vi "Find Path with Astar.vi"(8 "error in (no error)":errorcluster, 9 "goal node":cluster{"X":i32, "Y":i32}={"X"=32, "Y"=32}, 10 "start node":cluster{"X":i32, "Y":i32}={"X"=3, "Y"=3}, 11 "map reference in":refnum<data-value>) -> (1 "error out":errorcluster, 2 "intensity values":dbl[][](array[numeric]), 3 "map reference out":refnum<data-value>, 4 "y coordinates":i32[](array[numeric]), 6 "x coordinates":i32[](array[numeric]))   [LabVIEW 2017]
uses:
  <vilib>/robotics/Navigation/shared/WorldMap/OccupancyGridWorldMap/NI_Robotics_OccupancyGridWorldMap.lvclass
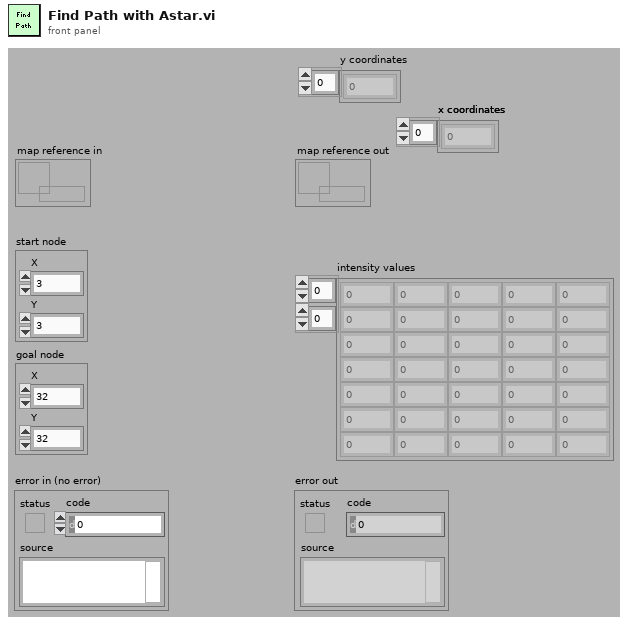
[diagram p1: front panel]
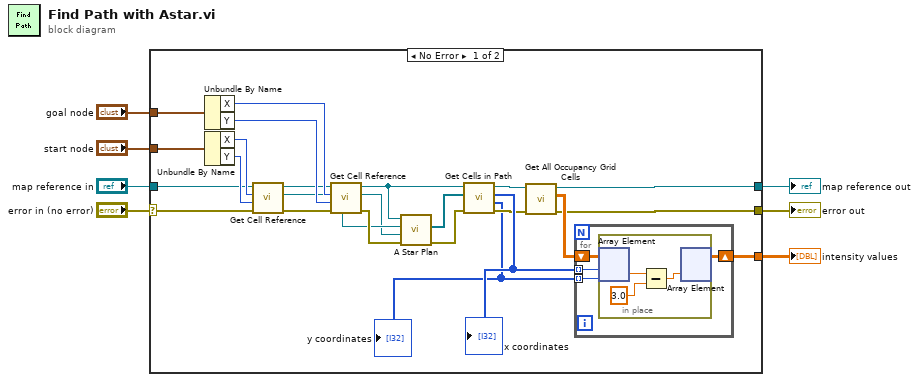
[diagram p0: block diagram]
diagram:
  n1 = case shown="No Error" "error in (no error)" {
    selector: "error in (no error)" -> [w14 w39]
    tunnel: "map reference in" -> [w15 w40]
    tunnel: "goal node" -> [w13 _]
    tunnel: "start node" -> [w12 _]
    tunnel: [w11 _] -> w3
    tunnel: [w10 w40] -> w2
    tunnel: [w9 w39] -> w1
    frame No Error {
      n2 = Unbundle By Name(w13) -> ("X"=w30:i32, "Y"=w31:i32)
      n3 = Unbundle By Name(w12) -> ("X"=w28:i32, "Y"=w29:i32)
      n4 = call <vilib>:"Get Cell Reference.vi"("error in (no error)"=w14, "y"=w29, "x"=w28, "map reference in"=w15) -> ("error out"=w19:errorcluster, "cell reference"=w17:refnum<data-value>, "map reference out"=w23:refnum<data-value>)  [unwired: 4 in, 1 out]
      n5 = call <vilib>:"Get Cell Reference.vi"("error in (no error)"=w19, "y"=w31, "x"=w30, "map reference in"=w23) -> ("error out"=w24:errorcluster, "cell reference"=w16:refnum<data-value>, "map reference out"=w21:refnum<data-value>)  [unwired: 4 in, 1 out]
      n6 = call <vilib>:"A Star Plan.vi"("error in (no error)"=w24, "goal reference"=w16, "start reference"=w17, "map reference in"=w21) -> ("error out"=w25:errorcluster, "path references"=w22:refnum<data-value>[])  [unwired: 4 in, 2 out]
      n7 = call <vilib>:"Get Cells in Path.vi"("error in (no error)"=w25, "path references"=w22, "map reference in"=w21) -> ("error out"=w18:errorcluster, "y coordinates"=w8:i32[], "x coordinates"=w27:i32[], "map reference out"=w20:refnum<data-value>)  [unwired: 5 in]
      "y coordinates" <- w8
      "x coordinates" <- w27
      n8 = call <vilib>:"Get All Occupancy Grid Cells.vi"("error in (no error)"=w18, "map reference in"=w20) -> ("error out"=w9:errorcluster, "occupancy grid"=w26:dbl[][], "map reference out"=w10:refnum<data-value>)  [unwired: 7 in]
      n9 = for {
        tunnel: w8 -> [w33] mode=indexing
        tunnel: w27 -> [w34] mode=indexing
        shift-right: [w32] -> w11
        shift-left: w26 -> [w35]
        n10 = in-place {
          n11 = in-place-array #1(w35, w34, w33) -> (w37:dbl)
          n12 = Subtract(x=w37, y=3.0) -> (x-y=w36:dbl)
          n13 = in-place-array #1(w36) -> (w32:dbl[][])  [unwired: 2 out]
        }
      }
    }
    frame Error {
    }
  }
  "error out" <- w1
  "intensity values" <- w3
  "map reference out" <- w2
